vi "EminemExecute.vi"(8 "error in (no error)":errorcluster) -> (0 "error out":errorcluster)   [LabVIEW 2023]
panel:
  # "Click here to set min"
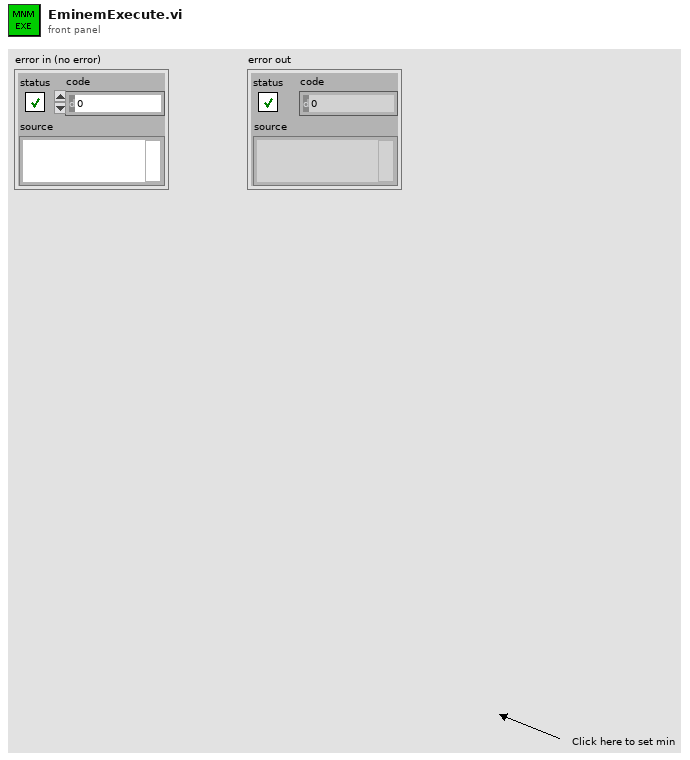
[diagram p1: front panel]
types:
  T1 = typedef "WPI_DigitalInputDevRef.ctl" = cluster{"DevStatus":errorcluster, "DIO Channel":T2}
  T2 = typedef "FPGA_DIOChannel.ctl" = enum8{"DIO 0", "DIO 1", "DIO 2", "DIO 3", "DIO 4", "DIO 5", "DIO 6", "DIO 7", "DIO 8", "DIO 9", "DIO MXP 0", "DIO MXP 1", "DIO MXP 2", "DIO MXP 3", "DIO MXP 4", "DIO MXP 5", "DIO MXP 6", "DIO MXP 7", "DIO MXP 8", "DIO MXP 9", "DIO MXP 10", "DIO MXP 11", "DIO MXP 12", "DIO MXP 13", "DIO MXP 14", "DIO MXP 15", "SPI Port CS1", "SPI Port CS2", "SPI Port CS3", "SPI Port MISO", "SPI Port MOSI", "Invalid"}
  T3 = typedef "WPI_MotorControlDeviceRef.ctl" = cluster{"DeviceStatus":errorcluster, "Type":T4, "PWM":cluster{"PWM Channel":T5, "DeadBand":T6}, "CAN":cluster{"Device Number":u8, "SetOutput VI Ref":variant, "GetOutput VI Ref":variant, "Enable VI Ref":variant, "Disable VI Ref":variant, "Data":variant}, "Invert":bool, "DIO PWM":cluster{"PWM \"Enable\" Channel":T5, "DIOChannel":T2, "PWM Rate":dbl}}
  T4 = typedef "WPI_MotorControlType.ctl" = enum16{"PWM", "CAN", "DIO PWM"}
  T5 = typedef "FPGA_DIOPWMChannel.ctl" = enum8{"PWM 0", "PWM 1", "PWM 2", "PWM 3", "PWM 4", "PWM 5", "PWM 6", "PWM 7", "PWM 8", "PWM 9", "PWM MXP 0", "PWM MXP 1", "PWM MXP 2", "PWM MXP 3", "PWM MXP 4", "PWM MXP 5", "PWM MXP 6", "PWM MXP 7", "PWM MXP 8", "PWM MXP 9", "Invalid"}
  T6 = typedef "WPI_PWMDeadband.ctl" = cluster{"Name":string, "maxPositivePwm":i32, "minPositivePwm":i32, "centerPwm":i32, "maxNegativePwm":i32, "minNegativePwm":i32, "angularRange":u16}
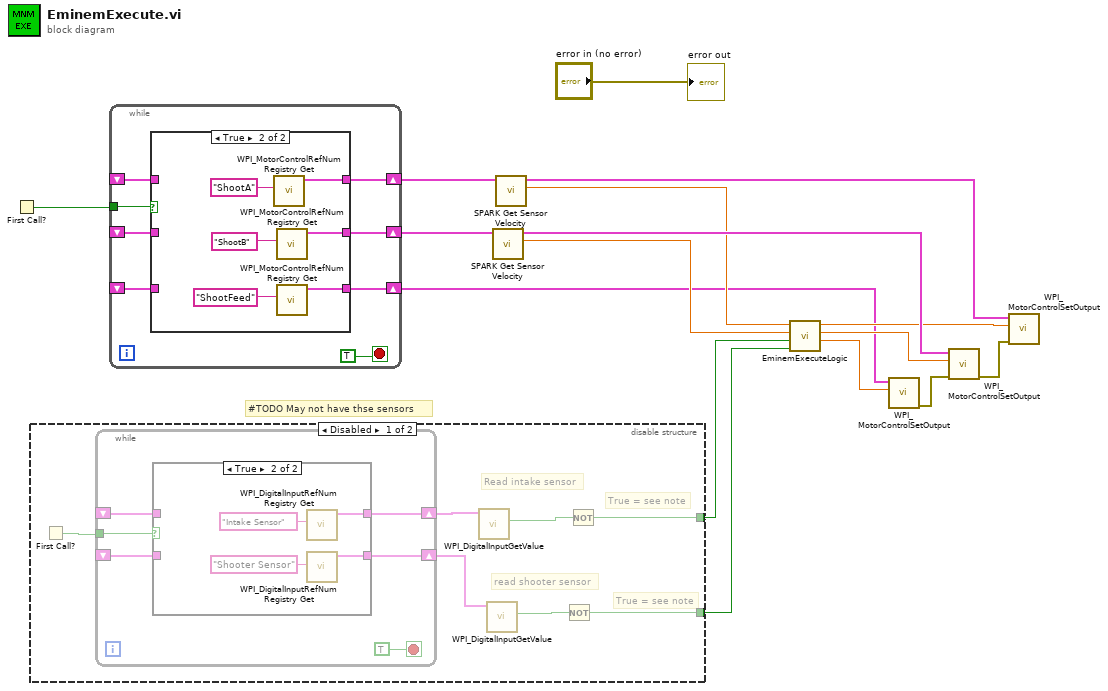
[diagram p0: block diagram]
diagram:
  # "#TODO May not have thse sensors"
  n1 = First Call?() -> (First Call?: T/F=w11:bool)
  n2 = disable-structure shown="Disabled" {
    disable-tunnel: [w18 _] -> w4
    disable-tunnel: [w17 _] -> w2
    frame Disabled {
      # "True = see note"
      # "True = see note"
      # "read shooter sensor"
      # "Read intake sensor"
      n3 = First Call?() -> (First Call?: T/F=w19:bool)
      n4 = while {
        tunnel: w19 -> [w27]
        shift-right: [w28] -> w22
        shift-left: _ -> [w26]
        shift-right: [w29] -> w23
        shift-left: _ -> [w25]
        stop <- TRUE stop-if-true
        n5 = case shown="True" w27 {
          tunnel: [w30 w35] -> w29
          tunnel: [w31 w34] -> w28
          tunnel: w26 -> [w31 _]
          tunnel: w25 -> [w30 _]
          frame False {
          }
          frame True {
            n6 = call <vilib>:"WPI_DigitalInputRefNum Registry Get.vi"("refnum name"="Intake Sensor") -> ("DigitalInputDevRef"=w34:T1)  [unwired: 9 in, 1 out]
            n7 = call <vilib>:"WPI_DigitalInputRefNum Registry Get.vi"("refnum name"="Shooter Sensor") -> ("DigitalInputDevRef"=w35:T1)  [unwired: 9 in, 1 out]
          }
        }
      }
      n8 = call <vilib>:"WPI_DigitalInputGetValue.vi"("DigitalInputDevRef"=w22) -> ("Value"=w21:bool)  [unwired: 8 in, 2 out]
      n9 = call <vilib>:"WPI_DigitalInputGetValue.vi"("DigitalInputDevRef"=w23) -> ("Value"=w20:bool)  [unwired: 8 in, 2 out]
      n10 = Not(x=w20) -> (.not. x?=w17:bool)
      n11 = Not(x=w21) -> (.not. x?=w18:bool)
    }
    frame Enabled {
    }
  }
  n12 = while {
    tunnel: w11 -> [w41]
    shift-right: [w43] -> w16
    shift-left: _ -> [w39]
    shift-right: [w42] -> w15
    shift-left: _ -> [w38]
    shift-right: [w37] -> w1
    shift-left: _ -> [w36]
    stop <- TRUE stop-if-true
    n13 = case shown="True" w41 {
      tunnel: [w46 w50] -> w43
      tunnel: [w45 w49] -> w42
      tunnel: w39 -> [w46 _]
      tunnel: w38 -> [w45 _]
      tunnel: [w44 w47] -> w37
      tunnel: w36 -> [w44 _]
      frame False {
      }
      frame True {
        n14 = call <vilib>:"WPI_MotorControlRefNum Registry Get.vi"("refnum name"="ShootA") -> ("MotorControlDevRef"=w50:T3)  [unwired: 9 in, 1 out]
        n15 = call <vilib>:"WPI_MotorControlRefNum Registry Get.vi"("refnum name"="ShootB") -> ("MotorControlDevRef"=w49:T3)  [unwired: 9 in, 1 out]
        n16 = call <vilib>:"WPI_MotorControlRefNum Registry Get.vi"("refnum name"="ShootFeed") -> ("MotorControlDevRef"=w47:T3)  [unwired: 9 in, 1 out]
      }
    }
  }
  n17 = call <vilib>:"SPARK Get Sensor Velocity.vi"("MotorControlDevRef in"=w15) -> ("Sensor Velocity"=w7:dbl, "MotorControlDevRef out"=w14:T3)  [unwired: 7 in, 2 out]
  n18 = call <vilib>:"SPARK Get Sensor Velocity.vi"("MotorControlDevRef in"=w16) -> ("Sensor Velocity"=w8:dbl, "MotorControlDevRef out"=w3:T3)  [unwired: 7 in, 2 out]
  n19 = call "EminemExecuteLogic.vi"("Ball Sensor B"=w2, "Ball Sensor A"=w4, "Shooter_B_Vel_RPM"=w7, "Shooter_A_Vel_RPM"=w8) -> ("Shooter_Feed_Motor_Out"=w12:dbl, "Shooter_B_Motor_Out"=w5:dbl, "Shooter_A_Motor_Out"=w6:dbl)  [unwired: 5 in]
  n20 = call <vilib>:"WPI_MotorControlSetOutput.vi"("Output"=w12, "MotorControlDevRef"=w1) -> ("error out"=w10:errorcluster)  [unwired: 7 in, 2 out]
  n21 = call <vilib>:"WPI_MotorControlSetOutput.vi"("error in (no error)"=w10, "Output"=w5, "MotorControlDevRef"=w14) -> ("error out"=w9:errorcluster)  [unwired: 6 in, 2 out]
  n22 = call <vilib>:"WPI_MotorControlSetOutput.vi"("error in (no error)"=w9, "Output"=w6, "MotorControlDevRef"=w3) -> ()  [unwired: 6 in, 3 out]
  "error out" <- "error in (no error)"
